vi "Pose2d_Interpolate.vi"(9 "T":dbl, 10 "EndValue Pose":T1 {"ROTATION"."SIN" format="%13.4f"; "ROTATION"."COS" format="%13.4f"; "ROTATION"."VALUE" format="%13.4f"; "TRANSLATION"."Y" format="%14.3f"; "TRANSLATION"."X" format="%14.3f"}, 11 "in POSE":T1 {"ROTATION"."SIN" format="%13.4f"; "ROTATION"."COS" format="%13.4f"; "ROTATION"."VALUE" format="%13.4f"; "TRANSLATION"."Y" format="%14.3f"; "TRANSLATION"."X" format="%14.3f"}) -> (3 "Interpolated Pose":T1={"TRANSLATION"={"X"=0.0, "Y"=0.0}, "ROTATION"={"VALUE"=0.0, "COS"=1.0, "SIN"=0.0}} {"ROTATION"."SIN" format="%13.4f"; "ROTATION"."COS" format="%13.4f"; "ROTATION"."VALUE" format="%13.4f"; "TRANSLATION"."Y" format="%14.3f"; "TRANSLATION"."X" format="%14.3f"})   [LabVIEW 2019, in "Trajectory_Library.lvlib"]
doc: "Interpolate between 2 poses\n\nParameter:\n - IN POSE - Current POSE data structure\n - EndValue POSE -- The end value POSE..\n - T -- Value between 0 and 1. \n\nReturns:\n - Interpolated POSE - The interpolated POSE."
uses:
  Trajectory_Library.lvlib
  POSE2D.ctl
  TRANSLATION2D.ctl
  ROTATION2D.ctl
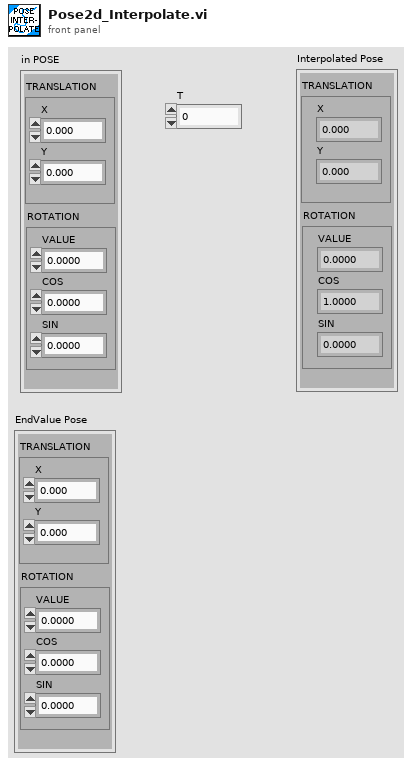
[diagram p1: front panel]
types:
  T1 = typedef "Trajectory_Library.lvlib/POSE2D.ctl" = cluster{"TRANSLATION":T2, "ROTATION":T3}
  T2 = typedef "Trajectory_Library.lvlib/TRANSLATION2D.ctl" = cluster{"X":dbl, "Y":dbl}
  T3 = typedef "Trajectory_Library.lvlib/ROTATION2D.ctl" = cluster{"VALUE":dbl, "COS":dbl, "SIN":dbl}
  T4 = typedef "Trajectory_Library.lvlib/TWIST2D.ctl" = cluster{"dX":dbl, "dY":dbl, "dTHETA":dbl}
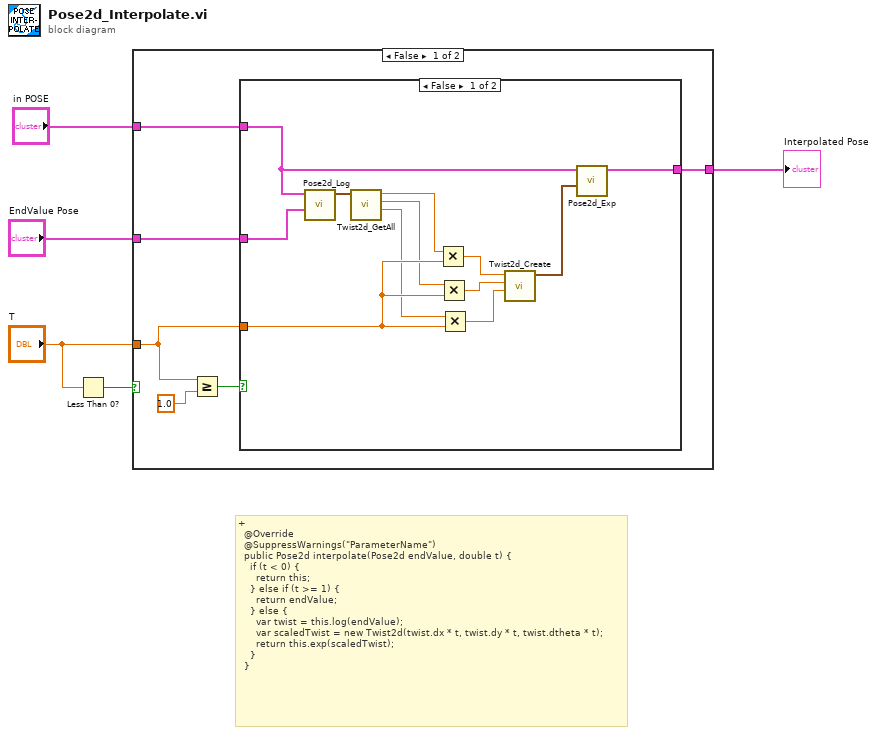
[diagram p0: block diagram]
diagram:
  # "+\n  @Override\n  @SuppressWarnings(\"ParameterName\")\n  public Pose2d interpolate(Pose2d endValue, double t) {\n    if (t < 0) {\n      return this;\n    } else if (t >= 1) {\n      return endValue;\n    } else {\n      var twist = this.log(endValue);\n      var scaledTwist = new Twist2d(twist.dx * t, twist.dy * t, twist.dtheta * t);\n      return this.exp(scaledTwist);\n    }\n  }"
  n1 = Less Than 0?(x="T") -> (x < 0?=w5:bool)
  n2 = case shown="False" w5 {
    tunnel: "T" -> [w6 _]
    tunnel: [w8 w25] -> w3
    tunnel: "in POSE" -> [w7 w25]
    tunnel: "EndValue Pose" -> [w9 _]
    frame False {
      n3 = Greater Or Equal?(x=w6, y=1.0) -> (x >= y?=w10:bool)
      n4 = case shown="False" w10 {
        tunnel: w9 -> [w23 w24]
        tunnel: [w12 w24] -> w8
        tunnel: w7 -> [w14 _]
        tunnel: w6 -> [w21 _]
        frame False {
          n5 = call "Pose2d_Log.vi"("end POSE"=w23, "in POSE"=w14) -> ("out TWIST"=w22:T4)  [unwired: 9 in]
          n6 = call "Twist2d_GetAll.vi"("TWIST"=w22) -> ("dTHETA"=w18:dbl, "dY"=w19:dbl, "dX"=w20:dbl)  [unwired: 8 in]
          n7 = Multiply(x=w20, y=w21) -> (x*y=w17:dbl)
          n8 = Multiply(x=w19, y=w21) -> (x*y=w16:dbl)
          n9 = Multiply(x=w18, y=w21) -> (x*y=w15:dbl)
          n10 = call "Twist2d_Create.vi"("dTHETA"=w15, "dY"=w16, "dX"=w17) -> ("TWIST"=w13:T4)  [unwired: 8 in]
          n11 = call "Pose2d_Exp.vi"("TWIST"=w13, "POSE"=w14) -> ("UpdatedPose"=w12:T1)  [unwired: 9 in]
        }
        frame True {
        }
      }
    }
    frame True {
    }
  }
  "Interpolated Pose" <- w3
